vi "SetIcon.vi"() -> ()   [LabVIEW 2011]
panel:
  out "Numeric":i32
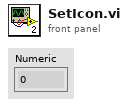
[diagram p1: front panel]
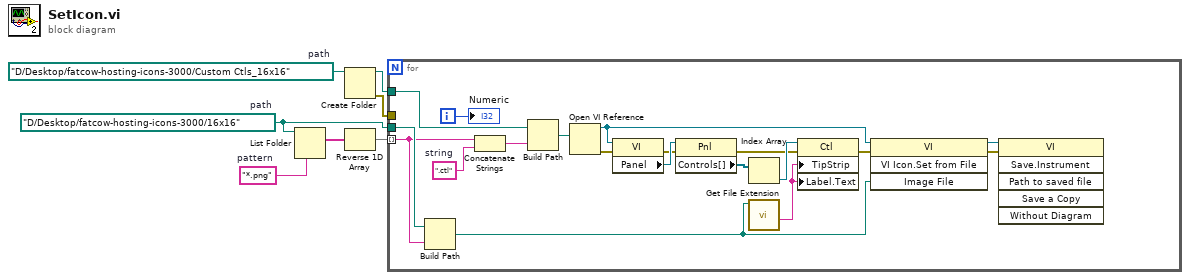
[diagram p0: block diagram]
diagram:
  w2 = path "D:/Desktop/fatcow-hosting-icons-3000/Custom Ctls_16x16"  # path
  w7 = "*.png"  # pattern
  w1 = path "D:/Desktop/fatcow-hosting-icons-3000/16x16"  # path
  n1 = List Folder(path=w1, pattern=w7) -> (filenames=w6:string[])  [unwired: 2 in, 3 out]
  n2 = Create Folder(path (use dialog)=w2) -> (created path=w5:path, error out=w4:errorcluster)  [unwired: 2 in, 1 out]
  n3 = Reverse 1D Array(array=w6) -> (reversed array=w3:string[])
  n4 = for {
    tunnel: w3 -> [w21] mode=indexing
    tunnel: w5 -> [w24]
    tunnel: w4 -> [_]
    tunnel: w1 -> [w22]
    i -> [w13]
    w26 = ".ctl"  # string
    n5 = Build Path(base path=w22, name or relative path=w21) -> (appended path=w15:path)
    n6 = Concatenate Strings(w21, w26) -> (w25:string)
    n7 = Build Path(base path=w24, name or relative path=w25) -> (appended path=w23:path)
    n8 = Open VI Reference(vi path=w23) -> (vi reference=w19:refnum<vi>, error out=w9:errorcluster)  [unwired: 5 in]
    n9 = property class="VI"(reference=w19, error in=w9) -> (error out=w12:errorcluster, "Panel"=w18:refnum<vi>)  [unwired: 1 out]
    n10 = property class="Pnl"(reference=w18, error in=w12) -> (error out=w11:errorcluster, "Controls[]"=w17:refnum<vi>[])  [unwired: 1 out]
    n11 = Index Array(array=w17) -> (element=w16:refnum<vi>)  [unwired: 1 in]
    n12 = call <vilib>:"Get File Extension.vi"("file"=w15) -> ("filename without extension"=w14:string)  [unwired: 7 in, 3 out]
    n13 = property class="Ctl"(reference=w16, error in=w11, "TipStrip"=w14, "Label.Text"=w14) -> (error out=w10:errorcluster)  [unwired: 1 out]
    n14 = invoke class="VI" method="VI Icon.Set from File"(reference=w19, error in=w10, "Image File"=w15) -> (reference out=w20:refnum<vi>, error out=w8:errorcluster)  [unwired: 1 in, 2 out]
    n15 = invoke class="VI" method="Save.Instrument"(reference=w20, error in=w8) -> ()  [unwired: 4 in, 6 out]
    "Numeric" <- w13
  }
